vi "Handle Data.vi"(8 "error in (no error)":errorcluster, 10 "Data":T1, 11 "Group Data Handler in":refnum<class "Group Data Handler.lvclass">) -> (0 "error out":errorcluster)   [LabVIEW 2020, in "VolatusHistorian.lvlib" / "Group Data Handler.lvclass"]
uses:
  Group Data Handler.lvclass
  Group Data Handler.lvclass/Group Data Handler.ctl
  Group Buffer DBL/Group Buffer DBL.lvclass
  lv-vecto/Vecto/Subscribed Data.ctl
  lv-vecto/Vecto/Vecto.lvlib
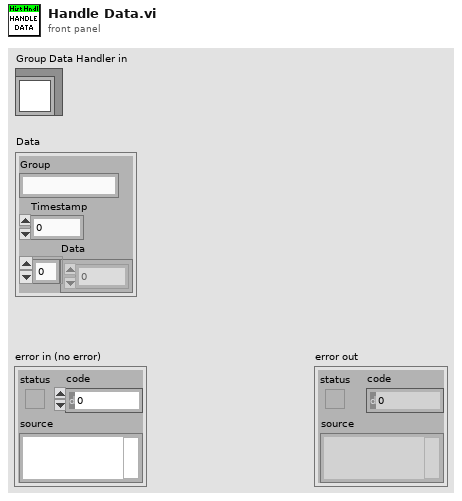
[diagram p1: front panel]
types:
  T1 = typedef "Vecto.lvlib/Subscribed Data.ctl" = cluster{"Group":string, "Timestamp":dbl, "Data":dbl[]}
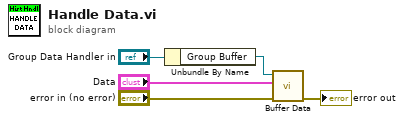
[diagram p0: block diagram]
diagram:
  n1 = Unbundle By Name("Group Data Handler in") -> ("Group Buffer"=w4:refnum<class "Group Buffer DBL.lvclass">)
  n2 = call "Buffer Data.vi"("error in (no error)"="error in (no error)", "Data"="Data", "Group Buffer DBL in"=w4) -> ("error out"=→"error out":errorcluster)  [unwired: 7 in, 1 out]
